vi "initFPGA.vi"() -> (2 "FPGA VI Reference Out":T1, 5 "error out":errorcluster)   [LabVIEW 2017]
uses:
  <vilib>/rvi/interface/nirviOpenFPGA/nirviOpenFPGA.xnode
  <vilib>/rvi/interface/nirviMethod/nirviMethod.xnode
  <vilib>/FPGAPlugInAG/cRIO-9118/niLvFpga_Run_cRIO-9118.vi
  FPGA Bitfiles/PVemulator_FPGATarget2_IpDFT-only-DC2x9_aEit3VyAdvg.lvbitx
  <vilib>/FPGAPlugInAG/cRIO-9118/niLvFpga_Open_cRIO-9118.vi
  FPGA Bitfiles/FPGA.ctl
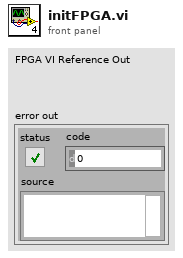
[diagram p1: front panel]
types:
  T1 = typedef "FPGA.ctl" = refnum<k20>
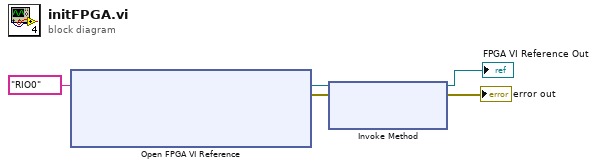
[diagram p0: block diagram]
diagram:
  n1 = xnode "Open FPGA VI Reference"("resource name"=tag "RIO0") -> ("FPGA VI Reference Out"=w1:T1, "error out"=w5:errorcluster)  [unwired: 1 in]
  n2 = xnode "Invoke Method"("FPGA VI Reference In"=w1, "error in"=w5) -> ("FPGA VI Reference Out"=→"FPGA VI Reference Out":T1, "error out"=→"error out":errorcluster)  [unwired: 1 in]
